vi "Recieve Pressure.vi"(8 "error in (no error)":errorcluster, 9 "ID":string, 10 "Pressure":dbl format="%#_13g", 11 "ADM.lvlib:ADM.lvclass":refnum<class "Main.lvclass">) -> (0 "error out":errorcluster, 3 "Actor out":refnum<class "Actor.lvclass">)   [LabVIEW 2018]
uses:
  Main.lvclass
  C:/Program Files (x86)/National Instruments/LabVIEW 2018/vi.lib/ActorFramework/Actor/Actor.lvclass
  <vilib>/ActorFramework/Actor/Actor.lvclass
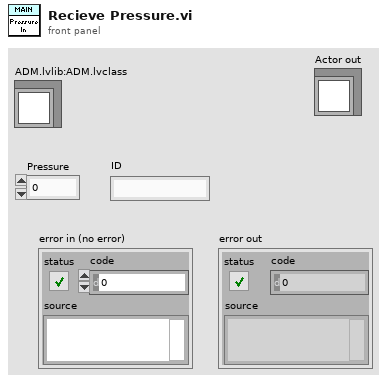
[diagram p1: front panel]
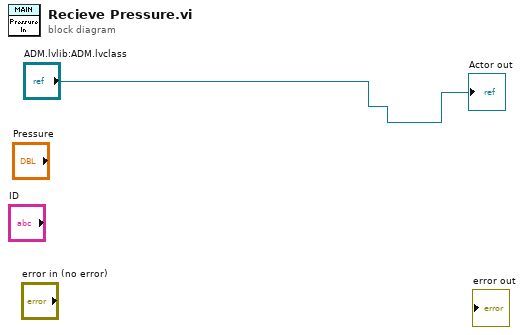
[diagram p0: block diagram]
diagram:
  "Actor out" <- "ADM.lvlib:ADM.lvclass"
